vi "Get Plugin Paths.vi"(0 "Measurement Customizations in":refnum<class "Measurement Customizations.lvclass">, 11 "error in (no error)":errorcluster) -> (4 "Measurement Customizations out":refnum<class "Measurement Customizations.lvclass">, 6 "Get Measurement Details VI Path":path, 8 "Measurement Logic VI Path":path, 10 "Measurement UI VI Path":path, 13 "Measurement Configuration CTL Path":path, 14 "Measurement Results CTL Path":path, 15 "error out":errorcluster)   [LabVIEW 2020, in "MeasurementLink Measurement Template.lvlib" / "Measurement Customizations.lvclass"]
uses:
  Measurement Customizations.lvclass
  Get Measurement Details.vi
  Measurement Logic.vi
  Measurement UI.vi
  Measurement Configuration.ctl
  Measurement Results.ctl
  Measurement Customizations.lvclass/Measurement Customizations.ctl
  MeasurementLink Measurement Template.lvlib
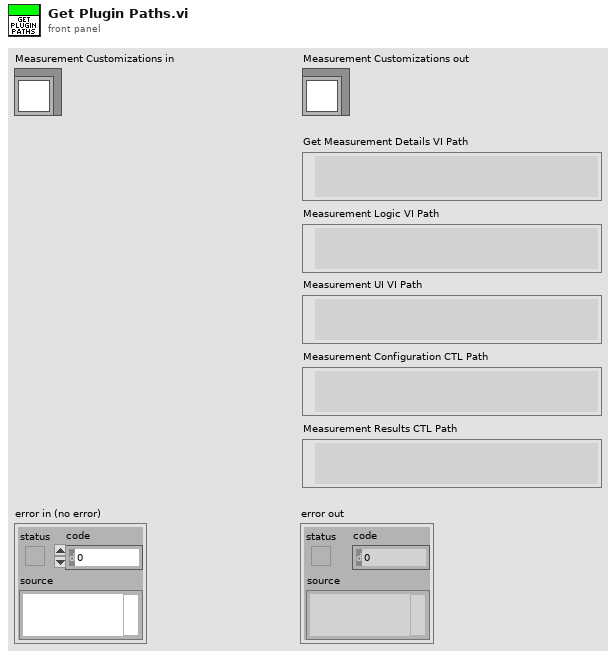
[diagram p1: front panel]
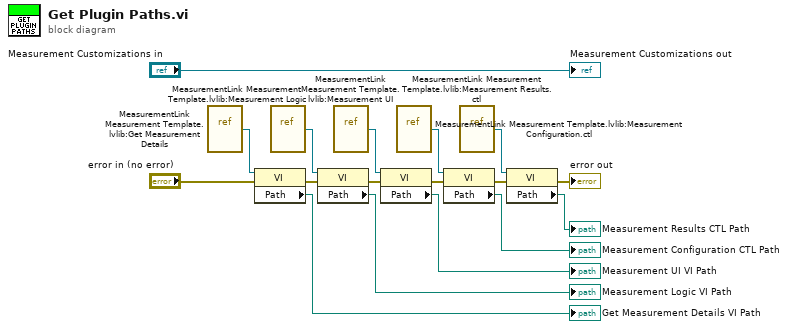
[diagram p0: block diagram]
diagram:
  n1 = vi-ref "MeasurementLink Measurement Template.lvlib:Get Measurement Details.vi"() -> (w1:refnum<vi>)
  n2 = property class="VI"(reference=w1, error in="error in (no error)") -> (error out=w6:errorcluster, "Path"=→"Get Measurement Details VI Path":path)  [unwired: 1 out]
  n3 = vi-ref "MeasurementLink Measurement Template.lvlib:Measurement Logic.vi"() -> (w14:refnum<vi>)
  n4 = property class="VI"(reference=w14, error in=w6) -> (error out=w5:errorcluster, "Path"=→"Measurement Logic VI Path":path)  [unwired: 1 out]
  n5 = vi-ref "MeasurementLink Measurement Template.lvlib:Measurement UI.vi"() -> (w12:refnum<vi>)
  n6 = property class="VI"(reference=w12, error in=w5) -> (error out=w4:errorcluster, "Path"=→"Measurement UI VI Path":path)  [unwired: 1 out]
  n7 = vi-ref "MeasurementLink Measurement Template.lvlib:Measurement Configuration.ctl"() -> (w10:refnum<vi>)
  n8 = property class="VI"(reference=w10, error in=w4) -> (error out=w3:errorcluster, "Path"=→"Measurement Configuration CTL Path":path)  [unwired: 1 out]
  n9 = vi-ref "MeasurementLink Measurement Template.lvlib:Measurement Results.ctl"() -> (w9:refnum<vi>)
  n10 = property class="VI"(reference=w9, error in=w3) -> (error out=→"error out":errorcluster, "Path"=→"Measurement Results CTL Path":path)  [unwired: 1 out]
  "Measurement Customizations out" <- "Measurement Customizations in"
